vi "8.4.vi"() -> ()   [LabVIEW 2017]
panel:
  out "Numeric 2":dbl
  out "Numeric":dbl
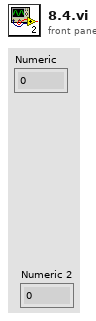
[diagram p1: front panel]
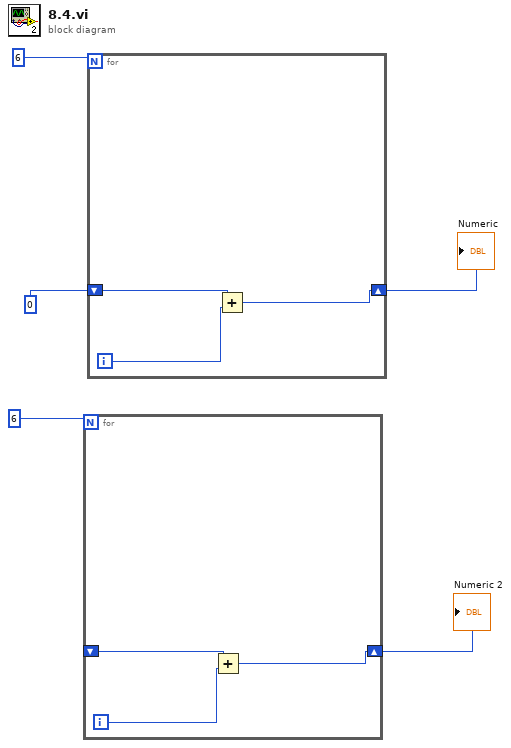
[diagram p0: block diagram]
diagram:
  n1 = for {
    N: 6 -> [_]
    shift-right: [w6] -> w1
    shift-left: _ -> [w8]
    i -> [w7]
    n2 = Add(x=w8, y=w7) -> (x+y=w6:i32)
  }
  "Numeric 2" <- w1
  n3 = for {
    N: 6 -> [_]
    shift-right: [w9] -> w3
    shift-left: 0 -> [w11]
    i -> [w10]
    n4 = Add(x=w11, y=w10) -> (x+y=w9:i32)
  }
  "Numeric" <- w3
